vi "WireReadTagbusVIs.vi"(5 "terminals data":refnum<vi>[](array[refnum]), 6 "DataTypes":T1[](array[typedef]), 7 "terminals indexes":refnum<vi>[](array[refnum]), 8 "error in":errorcluster, 9 "elements in cluster":i32, 10 "tag bus in in":refnum<vi>, 11 "VI in":refnum<vi>) -> (0 "error out":errorcluster, 2 "tag bus out":refnum<vi>, 3 "VI out":refnum<vi>)   [LabVIEW 2013]
uses:
  <vilib>/Utility/VariantDataType/Type.ctl
  <vilib>/Utility/miscctls.llb/LVPointTypeDef.ctl
  <vilib>/Utility/VariantDataType/VariantType.lvlib
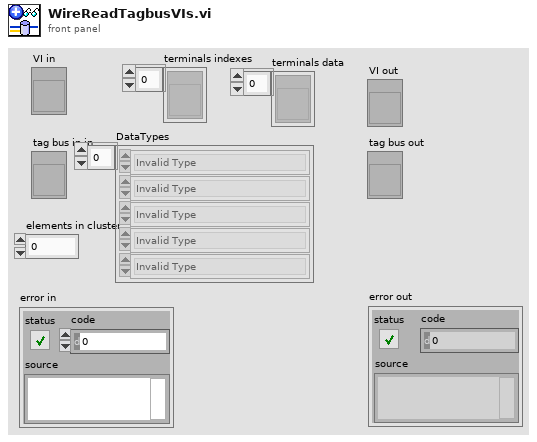
[diagram p1: front panel]
types:
  T1 = typedef "VariantType.lvlib/Type.ctl" = enum8{"Invalid Type", "Void", "I8", "I16", "I32", "I64", "U8", "U16", "U32", "U64", "Single Float", "Double Float", "Extended Float", "Single Complex", "Double Complex", "Extended Complex", "Enum U8", "Enum U16", "Enum U32", "Enum U64", "Single Float With Unit", "Double Float With Unit", "Extended Float With Unit", "Single Complex with Unit", "Double Complex with Unit", "Extended Complex with Unit", "Boolean", "String", "Path", "Picture", "Tag", "Array", "Cluster", "Variant", "LV Variant", "Waveform", "Timestamp", "Digital Waveform", "Digital Data", "ExpressData", "Refnum", "External Data", "VI", "Poly VI", "LabVIEW Class Instance", "Fixed Point"}
  T2 = typedef "LVPointTypeDef.ctl" = cluster{"Horizontal":i16, "Vertical":i16}
  T3 = typedef "tag bus.lvlib/tag descriptor.lvclass/Data Type.ctl" = enum16{"Double", "Single", "I64", "I32", "I16", "I8", "U64", "U32", "U16", "U8", "Boolean", "String", "Array of Double", "Array of Single", "Array of I64", "Array of I32", "Array of I16", "Array of I8", "Array of U64", "Array of U32", "Array of U16", "Array of U8", "Array of Boolean", "Array of String"}
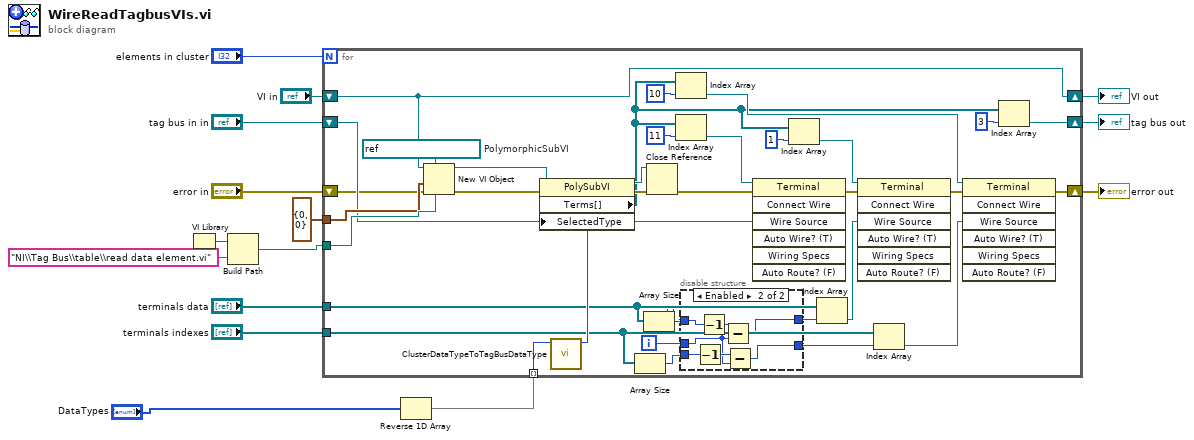
[diagram p0: block diagram]
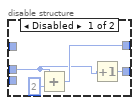
[diagram p2: hidden frame]
diagram:
  n1 = VI Library() -> (path=w3:path)
  n2 = Build Path(base path=w3, name or relative path="NI\\Tag Bus\\table\\read data element.vi") -> (appended path=w1:path)
  n3 = Reverse 1D Array(array="DataTypes") -> (reversed array=w4:T1[])
  n4 = for {
    N: "elements in cluster" -> [_]
    tunnel: w1 -> [w49]
    tunnel: T2 {"Horizontal"=0, "Vertical"=0} ("location") -> [w48]
    tunnel: "terminals data" -> [w19]
    tunnel: "terminals indexes" -> [w17]
    shift-right: [w33] -> w13
    shift-left: "tag bus in in" -> [w36]
    shift-right: [w32] -> w12
    shift-left: "VI in" -> [w32]
    shift-right: [w28] -> w6
    shift-left: "error in" -> [w27]
    tunnel: w4 -> [w23] mode=indexing
    i -> [w21]
    w47 = refnum<vi> refnum  # PolymorphicSubVI
    n5 = New VI Object(vi object class=w47, owner refnum=w32, position/next to=w48, 6:w49, 8:w27) -> (object refnum=w42:refnum<vi>, 0:w26:errorcluster)  [unwired: 3 in]
    n6 = call "ClusterDataTypeToTagBusDataType.vi"("Type Enum"=w23) -> ("data type"=w22:T3)  [unwired: 10 in]
    n7 = property on="Property Node" class="PolySubVI"(reference=w42, error in=w26, "SelectedType"=w22) -> (reference out=w44:refnum<vi>, error out=w43:errorcluster, "Terms[]"=w31:refnum<vi>[])
    n8 = Array Size(array=w17) -> (size(s)=w16:i32)
    n9 = Array Size(array=w19) -> (size(s)=w18:i32)
    n10 = Close Reference(reference=w44, error in (no error)=w43) -> (error out=w25:errorcluster)
    n11 = Index Array(array=w31, index=10) -> (element=w39:refnum<vi>)
    n12 = Index Array(array=w31, index=11) -> (element=w35:refnum<vi>)
    n13 = disable-structure shown="Enabled" {
      disable-tunnel: [w53 w60] -> w24
      disable-tunnel: w21 -> [w51 w55]
      disable-tunnel: [w50 w54] -> w20
      disable-tunnel: w18 -> [_ w59]
      disable-tunnel: w16 -> [_ w57]
      frame Disabled {
        n14 = Add(x=w51, y=2) -> (x+y=w53:i32)
        n15 = Increment(x=w51) -> (x+1=w50:i32)
      }
      frame Enabled {
        n16 = Decrement(x=w57) -> (x-1=w56:i32)
        n17 = Decrement(x=w59) -> (x-1=w58:i32)
        n18 = Subtract(x=w58, y=w55) -> (x-y=w60:i32)
        n19 = Subtract(x=w56, y=w55) -> (x-y=w54:i32)
      }
    }
    n20 = invoke on="Invoke Node" class="Terminal" method="Connect Wire"(reference=w35, error in=w25, "Wire Source"=w36) -> (error out=w30:errorcluster)  [unwired: 4 in, 6 out]
    n21 = Index Array(array=w31, index=1) -> (element=w41:refnum<vi>)
    n22 = Index Array(array=w19, index=w24) -> (element=w40:refnum<vi>)
    n23 = invoke on="Invoke Node" class="Terminal" method="Connect Wire"(reference=w41, error in=w30, "Wire Source"=w40) -> (error out=w29:errorcluster)  [unwired: 4 in, 6 out]
    n24 = Index Array(array=w17, index=w20) -> (element=w38:refnum<vi>)
    n25 = invoke on="Invoke Node" class="Terminal" method="Connect Wire"(reference=w39, error in=w29, "Wire Source"=w38) -> (error out=w28:errorcluster)  [unwired: 4 in, 6 out]
    n26 = Index Array(array=w31, index=3) -> (element=w33:refnum<vi>)
  }
  "tag bus out" <- w13
  "VI out" <- w12
  "error out" <- w6
